vi "ConnectedStatus.vi"(8 "error in (no error)":errorcluster, 11 "ChromaAcLoad in":refnum<class "ChromaAcLoad.lvclass">) -> (0 "error out":errorcluster, 2 "Any Connections?":bool, 3 "ChromaAcLoad out":refnum<class "ChromaAcLoad.lvclass">)   [LabVIEW 2018, in "AcPwrPlugins.lvlib" / "ChromaAcLoad.lvclass"]
doc: "This VI displays the boolean status of if the instrumetn is connected i.e. a valid reference to the instrument has been established."
uses:
  ChromaAcLoad.lvclass
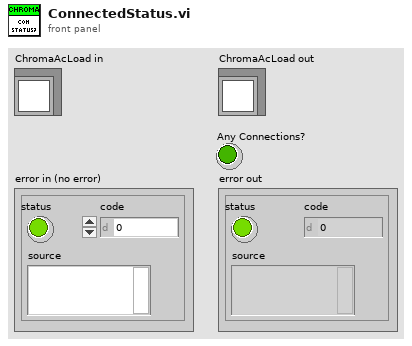
[diagram p1: front panel]
types:
  T1 = typedef "AcPwrPlugins.lvlib/ChromaAcLoad.lvclass/DeviceProperties.ctl" = cluster{"Frequency (Hz)":dbl, "Phases":cluster{"Handle":string, "Name":string, "Phase Select":i32, "SimulateInstrument(F)":bool, "id query (T)":bool, "reset device (T)":bool, "LC":cluster{"C (uF)":i32, "L (uH)":i32, "RS (Ohm)":dbl, "RL (Ohm)":dbl}, "Load Current (A/Arms)":dbl, "Load Voltage (V/Vrms)":dbl, "Load Power (W)":dbl, "Load Resistance (Ohms)":dbl, "Load Current Peak (A)":dbl, "Load Current Limit (A/Arms)":dbl, "Slew Rate":cluster{"Rise Slew Rate (Units/S)":i32, "Fall Slew Rate (Units/S)":i32}, "Load Short Circuited":bool, "Line Synchronization":bool, "Priority":enum16{"CF Only", "PF Only", "Both (CF)", "Both (PF)"}, "Crest Factor":dbl, "Power Factor":dbl, "Connected":bool, "Voltage Range (V)":dbl[], "Timing":cluster{"TimingOn":enum16{""}, "Hours":u32, "Minutes":u32, "Seconds":dbl, "CutoffVoltage":dbl}}[], "Configuration Mode":enum16{"Constant Voltage (DC)", "Constant Power (DC)", "Constant Power (AC)", "Constant Current (DC)", "Constant Current (AC)", "Constant Resistance (DC)", "Constant Resistance (AC)", "Rectified Mode (DC)", "Inrush (AC)", "RLC CP (AC)", "RLC (AC)"}}
  T2 = cluster{"Handle":string, "Name":string, "Phase Select":i32, "SimulateInstrument(F)":bool, "id query (T)":bool, "reset device (T)":bool, "LC":cluster{"C (uF)":i32, "L (uH)":i32, "RS (Ohm)":dbl, "RL (Ohm)":dbl}, "Load Current (A/Arms)":dbl, "Load Voltage (V/Vrms)":dbl, "Load Power (W)":dbl, "Load Resistance (Ohms)":dbl, "Load Current Peak (A)":dbl, "Load Current Limit (A/Arms)":dbl, "Slew Rate":cluster{"Rise Slew Rate (Units/S)":i32, "Fall Slew Rate (Units/S)":i32}, "Load Short Circuited":bool, "Line Synchronization":bool, "Priority":enum16{"CF Only", "PF Only", "Both (CF)", "Both (PF)"}, "Crest Factor":dbl, "Power Factor":dbl, "Connected":bool, "Voltage Range (V)":dbl[], "Timing":cluster{"TimingOn":enum16{""}, "Hours":u32, "Minutes":u32, "Seconds":dbl, "CutoffVoltage":dbl}}[]
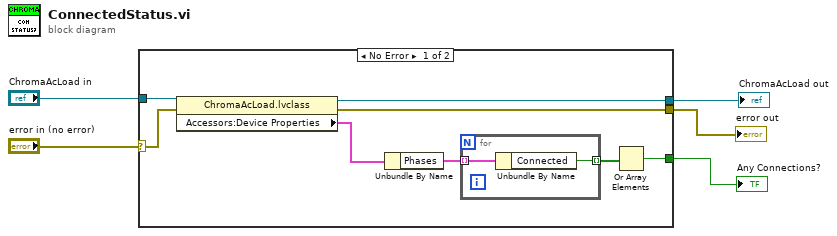
[diagram p0: block diagram]
diagram:
  n1 = case shown="No Error" "error in (no error)" {
    selector: "error in (no error)" -> [w12 w16]
    tunnel: "ChromaAcLoad in" -> [w13 w17]
    tunnel: [w11 w17] -> w3
    tunnel: [w9 w16] -> w2
    tunnel: [w8 _] -> w1
    frame No Error {
      n2 = property class="ChromaAcLoad.lvclass"(reference=w13, error in=w12) -> (reference out=w11:refnum<class "ChromaAcLoad.lvclass">, error out=w9:errorcluster, "Accessors:Device Properties"=w10:T1)
      n3 = Unbundle By Name(w10) -> ("Phases"=w7:T2)
      n4 = for {
        tunnel: w7 -> [w15] mode=indexing
        tunnel: [w14] -> w6 mode=indexing
        n5 = Unbundle By Name(w15) -> ("Connected"=w14:bool)
      }
      n6 = Or Array Elements(Boolean array=w6) -> (logical OR=w8:bool)
    }
    frame Error {
    }
  }
  "ChromaAcLoad out" <- w3
  "error out" <- w2
  "Any Connections?" <- w1
